vi "Close Chapter ref.vi"(0 "PDF Report IN":refnum<class "PDF Report Class.lvclass">, 11 "error in (no error)":errorcluster) -> (4 "PDF Report OUT":refnum<class "PDF Report Class.lvclass">, 15 "error out":errorcluster)   [LabVIEW 2019, in "Exaprom PDF.lvlib"]
doc: "Version 1.1\nDeveloped by Jean-Marc Simard\nCopyright © 2012, Exaprom Inc.\nAll rights reserved.\nLicense: BSD\n\nWith iTextSharp 4.1.6 (http://itextsharp.sourceforge.net)\nunder Mozilla Public License Version 1.1\n(http://www.mozilla.org/MPL/MPL-1.1.html)"
uses:
  LV Class/PDF Report Class/PDF Report Class.lvclass
  Exaprom PDF.lvlib
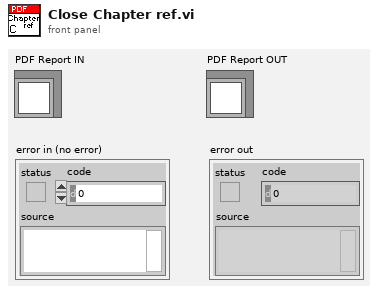
[diagram p1: front panel]
types:
  T1 = cluster{"ChapterAutoNumber":refnum<k24>, "Section [ ]":refnum<k24>[]}
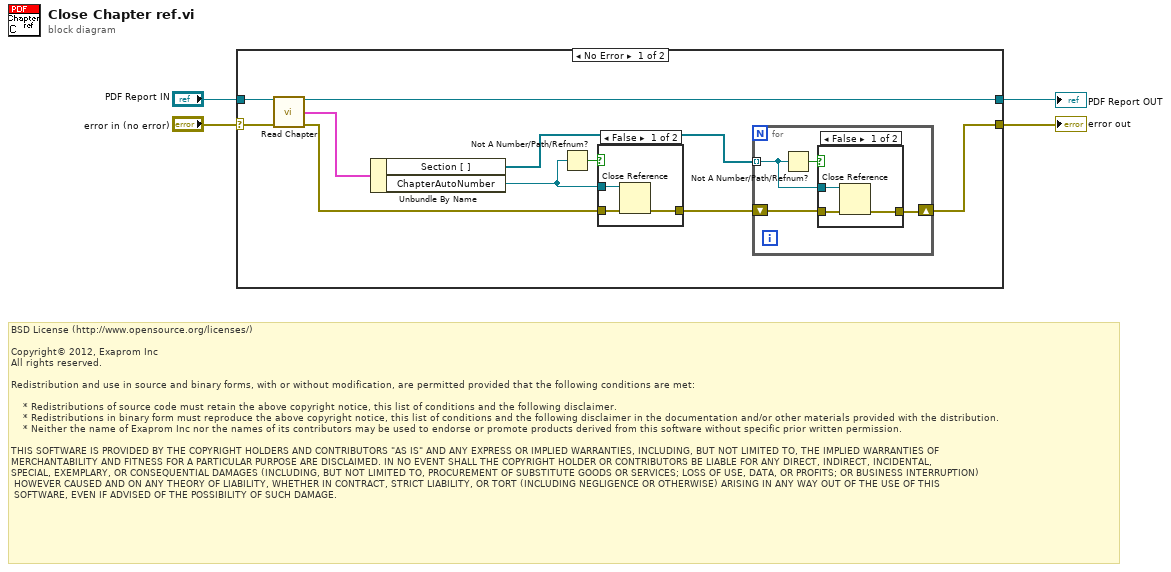
[diagram p0: block diagram]
diagram:
  # "BSD License (http://www.opensource.org/licenses/)\n\nCopyright© 2012, Exaprom Inc\nAll rights reserved.\n\nRedistribution and use in source and binary forms, with or without modification, are permitted provided that the following conditions are met:\n\n    * Redistributions of source code must retain the above copyright notice, this list of conditions and the following disclaimer.\n    * Redistributions in binary form must reproduce the above copyright notice, this list of conditions and the following disclaimer in the documentation and/or other materials provided with the distribution.\n    * Neither the name of Exaprom Inc nor the names of its contributors may be used to endorse or promote products derived from this software without specific prior written permission.\n\nTHIS SOFTWARE IS PROVIDED BY THE COPYRIGHT HOLDERS AND CONTRIBUTORS \"AS IS\" AND ANY EXPRESS OR IMPLIED WARRANTIES, INCLUDING, BUT NOT LIMITED TO, THE IMPLIED WARRANTIES OF \nMERCHANTABILITY AND FITNESS FOR A PARTICULAR PURPOSE ARE DISCLAIMED. IN NO EVENT SHALL THE COPYRIGHT HOLDER OR CONTRIBUTORS BE LIABLE FOR ANY DIRECT, INDIRECT, INCIDENTAL,\nSPECIAL, EXEMPLARY, OR CONSEQUENTIAL DAMAGES (INCLUDING, BUT NOT LIMITED TO, PROCUREMENT OF SUBSTITUTE GOODS OR SERVICES; LOSS OF USE, DATA, OR PROFITS; OR BUSINESS INTERRUPTION)\n HOWEVER CAUSED AND ON ANY THEORY OF LIABILITY, WHETHER IN CONTRACT, STRICT LIABILITY, OR TORT (INCLUDING NEGLIGENCE OR OTHERWISE) ARISING IN ANY WAY OUT OF THE USE OF THIS\n SOFTWARE, EVEN IF ADVISED OF THE POSSIBILITY OF SUCH DAMAGE."
  n1 = case shown="No Error" "error in (no error)" {
    selector: "error in (no error)" -> [w12 w28]
    tunnel: "PDF Report IN" -> [w14 w27]
    tunnel: [w13 w27] -> w3
    tunnel: [w6 w28] -> w2
    frame No Error {
      n2 = call-dynamic "Read Chapter.vi"("PDF Report Class in"=w14, "error in (no error)"=w12) -> ("PDF Report Class out"=w13:refnum<class "PDF Report Class.lvclass">, "Chapter ref"=w11:T1, "error out"=w8:errorcluster)  [unwired: 11 in]
      n3 = Unbundle By Name(w11) -> ("Section [ ]"=w5:refnum<k24>[], "ChapterAutoNumber"=w9:refnum<k24>)
      n4 = Not A Number/Path/Refnum?(number/path/refnum=w9) -> (NaN/Path/Refnum?=w10:bool)
      n5 = case shown="False" w10 {
        tunnel: w9 -> [w25 _]
        tunnel: w8 -> [w24 w26]
        tunnel: [w23 w26] -> w7
        frame False {
          n6 = Close Reference(reference=w25, error in (no error)=w24) -> (error out=w23:errorcluster)
        }
        frame True {
        }
      }
      n7 = for {
        shift-right: [w16] -> w6
        shift-left: w7 -> [w17]
        tunnel: w5 -> [w15] mode=indexing
        n8 = Not A Number/Path/Refnum?(number/path/refnum=w15) -> (NaN/Path/Refnum?=w18:bool)
        n9 = case shown="False" w18 {
          tunnel: w15 -> [w21 _]
          tunnel: w17 -> [w20 w22]
          tunnel: [w19 w22] -> w16
          frame False {
            n10 = Close Reference(reference=w21, error in (no error)=w20) -> (error out=w19:errorcluster)
          }
          frame True {
          }
        }
      }
    }
    frame Error {
    }
  }
  "PDF Report OUT" <- w3
  "error out" <- w2
